vi "new Server.vi"   [LabVIEW 2014]
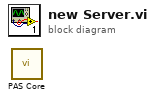
[diagram p0: block diagram]
diagram:
  n1 = call "PAS Core.vi"() -> ()  [unwired: 19 in, 1 out]
